vi "3.3 Building Virtual Instruments-Lab1(Prob1).vi"() -> ()   [LabVIEW 2025]
panel:
  in  "stop":bool
  out "Average":dbl
  out "Sum":dbl
  in  "Input  4":dbl
  in  "Input  3":dbl
  in  "Input 2":dbl
  in  "Input 1":dbl
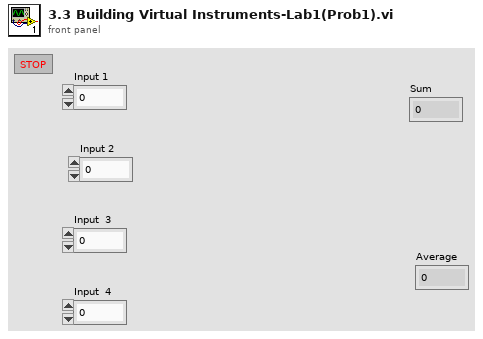
[diagram p1: front panel]
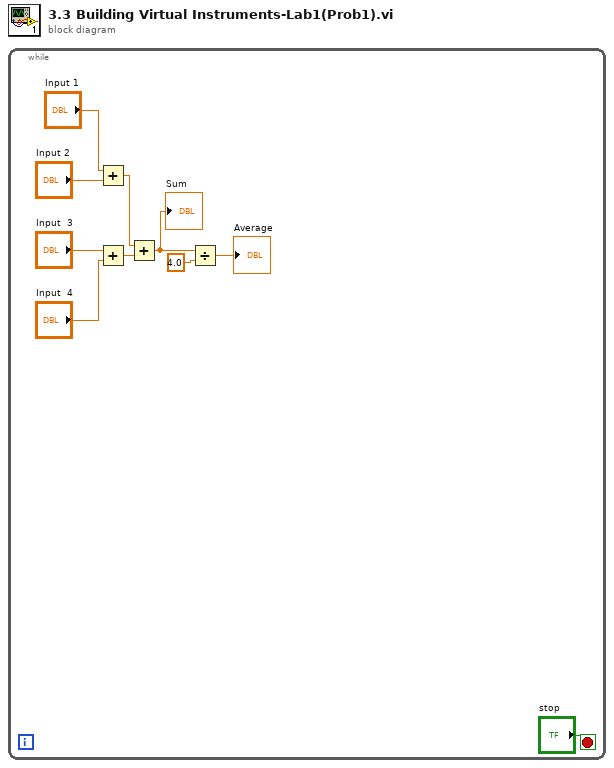
[diagram p0: block diagram]
diagram:
  n1 = while {
    stop <- "stop" stop-if-true
    n2 = Add(x="Input 1", y="Input 2") -> (x+y=w6:dbl)
    n3 = Add(x="Input  3", y="Input  4") -> (x+y=w5:dbl)
    n4 = Add(x=w6, y=w5) -> (x+y=w4:dbl)
    "Sum" <- w4
    n5 = Divide(x=w4, y=4.0) -> (x/y=→"Average":dbl)
  }
